vi "Test Local Queue Connection.vi"() -> ()   [LabVIEW 2013]
uses:
  MQTT_LocalQueue/Connection/LocalQueueConnection.lvclass
  MQTT_Connection/Connection/Connection.lvclass
panel:
  out "value":dbl
  out "listener error":errorcluster
  out "client session error":errorcluster
  out "server session error":errorcluster
  out "Bytes":u8[](array[numeric]) format="%08b"
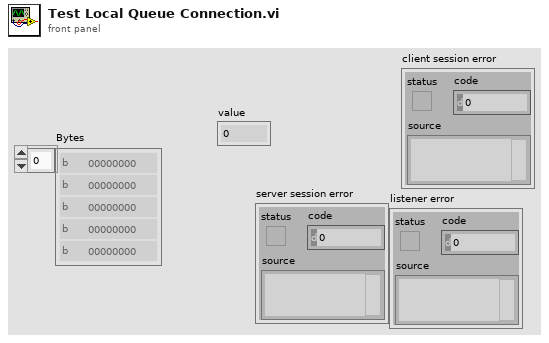
[diagram p1: front panel]
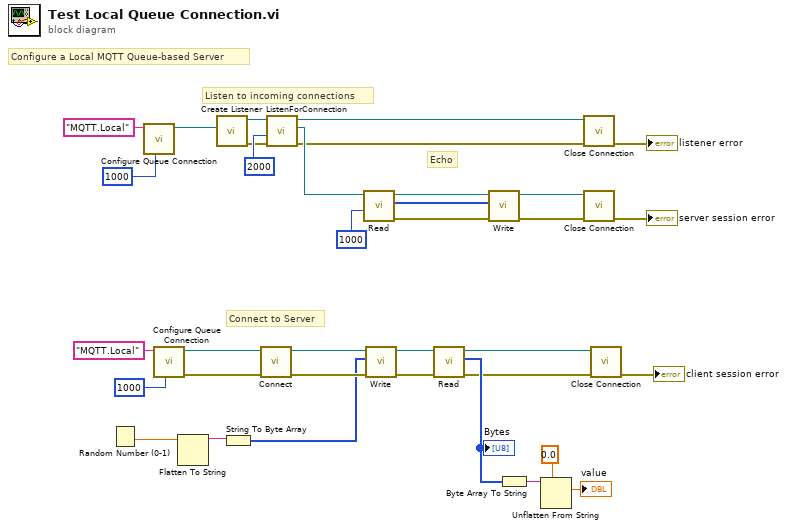
[diagram p0: block diagram]
diagram:
  # "Connect to Server"
  # "Echo"
  # "Listen to incoming connections"
  # "Configure a Local MQTT Queue-based Server"
  n1 = Random Number (0-1)() -> (number: 0 to 1=w15:dbl)
  n2 = call "Configure Queue Connection.vi"("timeout (500 ms)"=1000 ("timeout (100ms)"), "Queue Name"="MQTT.Local") -> ("LocalQueueConnection"=w30:refnum<class "LocalQueueConnection.lvclass">)  [unwired: 8 in, 1 out]
  n3 = call "Configure Queue Connection.vi"("timeout (500 ms)"=1000 ("timeout (100ms)"), "Queue Name"="MQTT.Local") -> ("error out"=w18:errorcluster, "LocalQueueConnection"=w24:refnum<class "LocalQueueConnection.lvclass">)  [unwired: 8 in]
  n4 = Flatten To String(anything=w15) -> (data string=w14:string)  [unwired: 3 in, 2 out]
  n5 = call "Create Listener.vi"("Connection Configuration"=w30) -> ("error out"=w31:errorcluster, "Listener"=w34:refnum<class "Connection.lvclass">)  [unwired: 9 in]
  n6 = String To Byte Array(string=w14) -> (unsigned byte array=w13:u8[])
  n7 = call "Connect.vi"("error in (no error)"=w18, "Connection in"=w24) -> ("error out"=w19:errorcluster, "Connection out"=w23:refnum<class "LocalQueueConnection.lvclass">)  [unwired: 8 in]
  n8 = call "ListenForConnection.vi"("error in (no error)"=w31, "timeout (ms)"=2000 ("bytes to read (100)"), "Listener"=w34) -> ("error out"=w6:errorcluster, "Connection"=w28:refnum<class "Connection.lvclass">, "Listener out"=w32:refnum<class "Connection.lvclass">)  [unwired: 5 in, 1 out]
  n9 = call "Read.vi"("timeout (1000 ms)"=1000 ("bytes to read (100)"), "TCPConnection in"=w28) -> ("error out"=w21:errorcluster, "Bytes"=w26:u8[], "TCPConnection out"=w27:refnum<class "Connection.lvclass">)  [unwired: 5 in, 2 out]
  n10 = call "Write.vi"("error in (no error)"=w19, "Bytes"=w13, "Connection in"=w23) -> ("error out"=w20:errorcluster, "Connection"=w22:refnum<class "LocalQueueConnection.lvclass">)  [unwired: 7 in]
  n11 = call "Read.vi"("error in (no error)"=w20, "TCPConnection in"=w22) -> ("error out"=w3:errorcluster, "Bytes"=w12:u8[], "TCPConnection out"=w1:refnum<class "LocalQueueConnection.lvclass">)  [unwired: 5 in, 2 out]
  "Bytes" <- w12
  n12 = call "Write.vi"("error in (no error)"=w21, "Bytes"=w26, "Connection in"=w27) -> ("error out"=w4:errorcluster, "Connection"=w16:refnum<class "Connection.lvclass">)  [unwired: 7 in]
  n13 = Byte Array To String(unsigned byte array=w12) -> (string=w11:string)
  n14 = Unflatten From String(type=0.0, binary string=w11) -> (value=→"value":dbl)  [unwired: 3 in, 2 out]
  n15 = call "Close Connection.vi"("error in (no error)"=w6, "Connection in"=w32) -> ("error out"=→"listener error":errorcluster)  [unwired: 8 in, 1 out]
  n16 = call "Close Connection.vi"("error in (no error)"=w4, "Connection in"=w16) -> ("error out"=→"server session error":errorcluster)  [unwired: 8 in, 1 out]
  n17 = call "Close Connection.vi"("error in (no error)"=w3, "Connection in"=w1) -> ("error out"=→"client session error":errorcluster)  [unwired: 8 in, 1 out]
